vi "test Import Configuration File (Sequential Use).vi"(8 "error in":errorcluster, 11 "TestCase in":refnum<class "Import.lvclass">) -> (0 "error out":errorcluster, 3 "TestCase out":refnum<class "Import.lvclass">)   [LabVIEW 2020, in "Import.lvclass"]
uses:
  Import.lvclass
  <vilib>/addons/_JKI Toolkits/VI Tester/TestCase.llb/TestCase.lvclass
  Import/ARINC 429 Import.lvlib
  <vilib>/NI/VeriStand Custom Device Testing Tools/VeriStandTestUtilities/VeriStandTestUtilities.lvlib
  C:/Program Files (x86)/National Instruments/LabVIEW 2020/vi.lib/addons/_JKI Toolkits/VI Tester/TestCase.llb/TestCase.lvclass
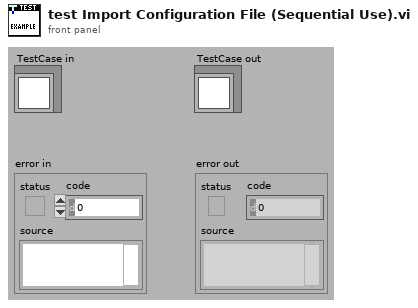
[diagram p1: front panel]
types:
  T1 = typedef "VS Channels Definition for All Labels on Hardware Channel.ctl" = cluster{"hardware channel":i32, "direction":T2, "labels":T3[], "speed":T8}
  T2 = typedef "Direction.ctl" = enum16{"Rx", "Tx"}
  T3 = typedef "VS Channels Definition for Label.ctl" = cluster{"label (Dec)":u32, "parameters":T4[], "SDI value":u8, "SDI enabled":bool, "transfer type":T7, "create timestamp":bool, "transmit period":u32}
  T4 = typedef "VS Channel Definition for Parameter.ctl" = cluster{"name":string, "unit":string, "Parameter":T5}
  T5 = typedef "Parameter Definition.ctl" = cluster{"start index":i32, "size":i32, "encoding":T6, "signed":bool, "scale multiplier":dbl, "scale offset":dbl, "default value":dbl}
  T6 = typedef "Encoding and Decoding.lvlib/Encoding.ctl" = enum16{"BNR", "BCD", "Discrete"}
  T7 = typedef "Transfer Type.ctl" = enum16{"Scheduled", "Acyclic", "Block", "Strobe"}
  T8 = typedef "Transfer Speed.ctl" = enum16{"LO (12.5 kb/s)", "HI (100 kb/s)"}
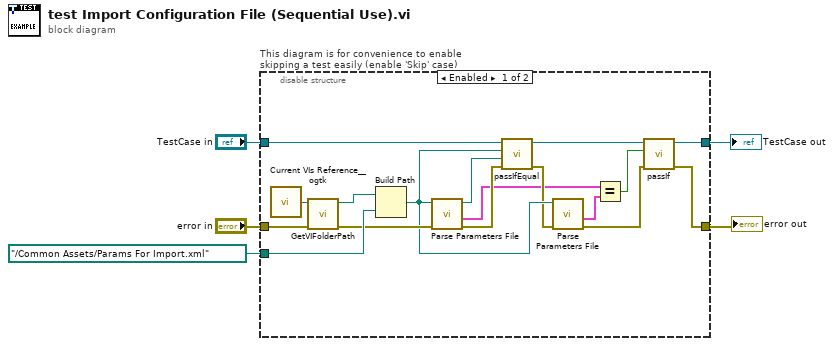
[diagram p0: block diagram]
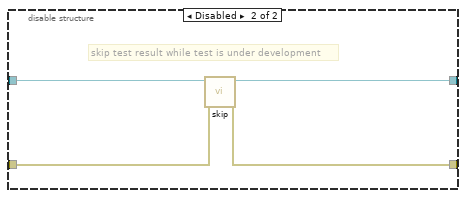
[diagram p2: hidden frame]
diagram:
  n1 = disable-structure "This diagram is for convenience to enable skipping a test easily (enable 'Skip' case)" shown="Enabled" {
    disable-tunnel: "TestCase in" -> [w22 w26]
    disable-tunnel: [w16 w24] -> w2
    disable-tunnel: [w17 w25] -> w4
    disable-tunnel: "error in" -> [w20 w23]
    disable-tunnel: path "../Common Assets/Params For Import.xml" ("Absolute or Relative Path") -> [w19 _]
    frame Enabled {
      n2 = call <userlib>:"Current VIs Reference__ogtk.vi"() -> ("Current VI's reference"=w21:refnum<vi>)  [unwired: 5 in]
      n3 = call <vilib>:"GetVIFolderPath.vi"("error in (no error)"=w20, "VI Reference in"=w21) -> ("error out"=w18:errorcluster, "VI Folder Path out"=w13:path)  [unwired: 8 in]
      n4 = Build Path(base path=w13, name or relative path=w19) -> (appended path=w14:path)
      n5 = call "Parse Parameters File.vi"("error in"=w18, "path to XML document"=w14) -> ("error out"=w12:errorcluster, "ports"=w7:T1[], "path to XML document out"=w8:path)  [unwired: 7 in]
      n6 = call-dynamic "passIfEqual.vi"("error in (no error)"=w12, "y"=w8, "x"=w14, "TestCase in"=w22) -> ("error out"=w10:errorcluster, "TestCase out"=w11:refnum<class "Import.lvclass">)  [unwired: 6 in]
      n7 = call "Parse Parameters File.vi"("error in"=w10, "path to XML document"=w14) -> ("error out"=w9:errorcluster, "ports"=w6:T1[])  [unwired: 7 in, 1 out]
      n8 = Equal?(x=w7, y=w6) -> (x = y?=w15:bool)
      n9 = call-dynamic "passIf.vi"("error in (no error)"=w9, "pass"=w15, "TestCase in"=w11) -> ("error out"=w17:errorcluster, "TestCase out"=w16:refnum<class "Import.lvclass">)  [unwired: 7 in]
    }
    frame Disabled {
      # "skip test result while test is under development"
      n10 = call <vilib>:"skip.vi"("error in (no error)"=w23, "TestCase in"=w26) -> ("error out"=w25:errorcluster, "TestCase out"=w24:refnum<class "Import.lvclass">)  [unwired: 8 in]
    }
  }
  "error out" <- w4
  "TestCase out" <- w2
